vi "PomiarTESTOWYpmp.vi"(3 "Wybór obiektu":u32(slide)=1 scale=1.0..4.0, 4 "WLACZ":bool, 5 "Liniowy/Logarytmiczny":bool, 6 "Amplituda":dbl, 7 "F min":dbl, 8 "ilosc probek":u32, 9 "F max":dbl) -> (0 "Czestotliwosc":dbl[](array[numeric]), 1 "V in":dbl[](array[numeric]), 2 "V out":dbl[](array[numeric]))   [LabVIEW 2021]
doc: "W tym SubVi dokonywany jest pomiar oraz wyliczanę są wymagane wartosci"
uses:
  <userlib>/Open_device_2018.llb/Select_Instr.ctl
panel:
  out "error out 3":errorcluster
  in  "error in (no error) 2":errorcluster
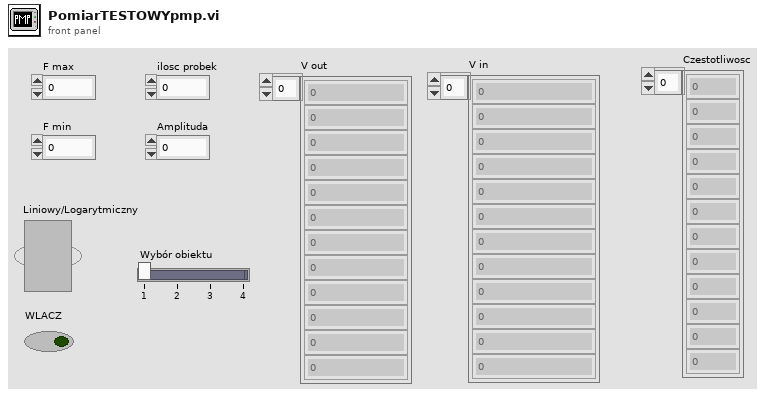
[diagram p1: front panel]
types:
  T1 = typedef "Select_Instr.ctl" = string
  T2 = cluster{"VISA resource name 1":refnum<visa-resource-name>, "VISA resource name 2":refnum<visa-resource-name>, "VISA resource name 3":refnum<visa-resource-name>}
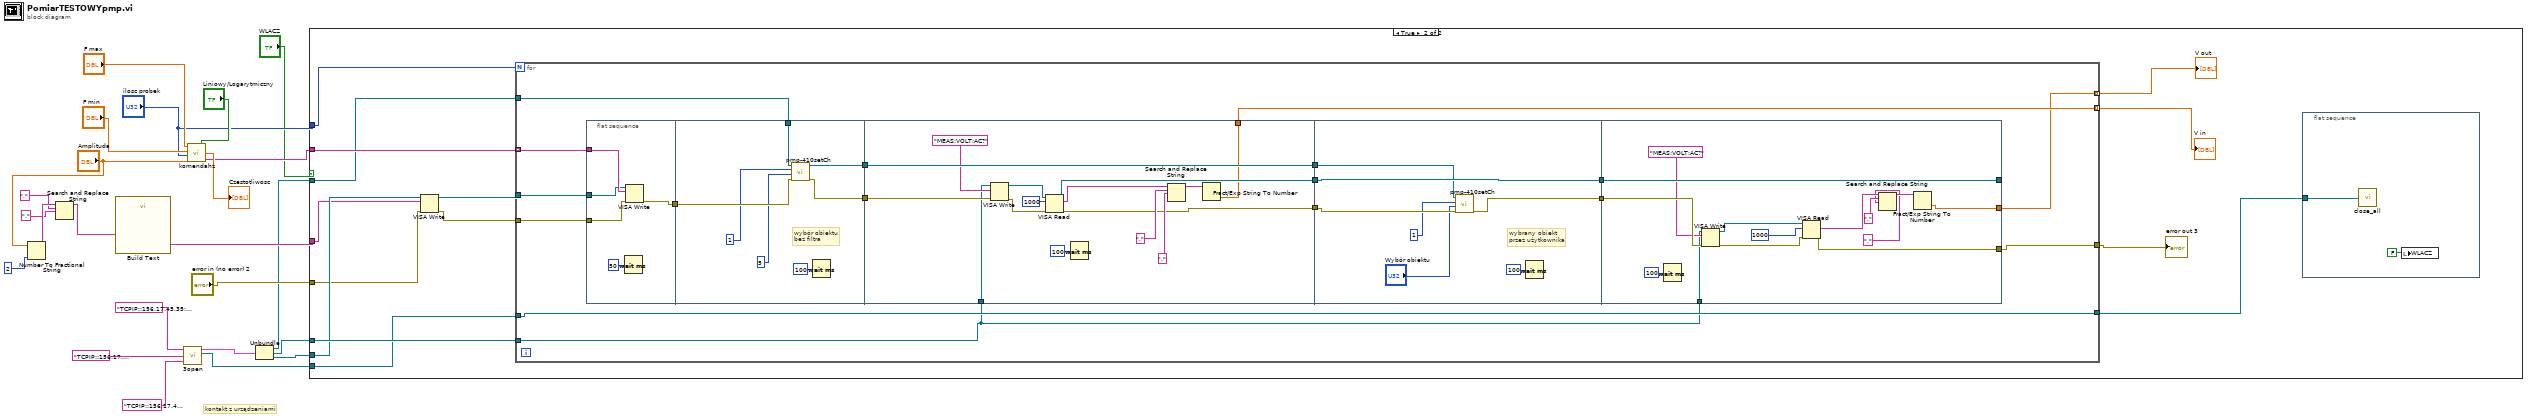
[diagram p0: block diagram]
diagram:
  # "kontakt z urządzeniami"
  n1 = Number To Fractional String(number="Amplituda", precision (6)=i16 2) -> (F-format string=w15:string)  [unwired: 2 in]
  n2 = Search and Replace String(input string=w15, search string=",", replace string="." ("replace string (\"\")")) -> (result string=w12:string)  [unwired: 5 in, 3 out]
  n3 = call "Build Text"("value"=w12) -> ("Result"=w9:string)  [unwired: 13 in, 1 out]
  n4 = call <userlib>:"3open.vi"("VISA resource name 1"=T1 "TCPIP::156.17.45.35::inst104::INSTR" ("Select_Instrument"), "VISA resource name 2"=T1 "TCPIP::156.17.45.35::inst27::INSTR" ("Select_Instrument"), "VISA resource name 3"=T1 "TCPIP::156.17.45.35::inst26::INSTR" ("Select_Instrument")) -> ("InstrCluster"=w5:T2, "InstrArray"=w2:refnum<visa-resource-name>[])  [unwired: 1 in, 2 out]
  n5 = call "komendahz.vi"("Liniowy/logarytmiczny"="Liniowy/Logarytmiczny", "Amplituda"="Amplituda", "ilosc probek"="ilosc probek", "F min"="F min", "F max"="F max") -> ("komendy"=w17:string[], "Czestotliwosci"=→"Czestotliwosc":dbl[])
  n6 = Unbundle(w5) -> ("VISA resource name 1"=w1:refnum<visa-resource-name>, "VISA resource name 2"=w3:refnum<visa-resource-name>, "VISA resource name 3"=w4:refnum<visa-resource-name>)
  n7 = case shown="True" "WLACZ" {
    tunnel: "ilosc probek" -> [_ w37]
    tunnel: "error in (no error) 2" -> [_ w28]
    tunnel: w17 -> [_ w36]
    tunnel: w9 -> [_ w29]
    tunnel: w4 -> [_ w30]
    tunnel: w3 -> [_ w33]
    tunnel: w2 -> [_ w25]
    tunnel: w1 -> [_ w32]
    frame False {
    }
    frame True {
      n8 = VISA Write(VISA resource name=w30, write buffer=w29, error in (no error)=w28) -> (VISA resource name out=w24:refnum<visa-resource-name>, error out=w27:errorcluster)  [unwired: 1 out]
      n9 = for {
        N: w37 -> [_]
        tunnel: w36 -> [w55] mode=indexing
        tunnel: [w41] -> w35 mode=indexing
        tunnel: [w48] -> w34 mode=indexing
        tunnel: w27 -> [w54]
        tunnel: w33 -> [w40]
        tunnel: w32 -> [w51]
        tunnel: [w56] -> w31
        tunnel: w25 -> [w56]
        tunnel: [w42] -> w26
        tunnel: w24 -> [w53]
        n10 = flat-sequence {
          tunnel: w55 -> [w61]
          tunnel: w54 -> [w60]
          tunnel: w53 -> [w58]
          tunnel: [w59] -> w52
          tunnel: w52 -> [w68]
          tunnel: w51 -> [w65]
          tunnel: [w64] -> w50
          tunnel: [w63] -> w49
          tunnel: w50 -> [w77]
          tunnel: w49 -> [w83]
          tunnel: w40 -> [w75]
          tunnel: [w70] -> w48
          tunnel: [w83] -> w47
          tunnel: [w72] -> w46
          tunnel: [w71] -> w45
          tunnel: w47 -> [w87]
          tunnel: w46 -> [w89]
          tunnel: w45 -> [w90]
          tunnel: [w90] -> w44
          tunnel: [w86] -> w43
          tunnel: [w104] -> _
          tunnel: w44 -> [w104]
          tunnel: w43 -> [w98]
          tunnel: [w94] -> w42
          tunnel: [w93] -> w41
          tunnel: w40 -> [w91]
          frame #0 {
            n11 = Wait (ms)(milliseconds to wait=u32 50) -> ()  [unwired: 1 out]
            n12 = VISA Write(VISA resource name=w58, write buffer=w61, error in (no error)=w60) -> (error out=w59:errorcluster)  [unwired: 2 out]
          }
          frame #1 {
            # "wybór obiektu\nbez filtra"
            n13 = call <userlib>:"pmp-410setCh.vi"("error in (no error)"=w68, "Channel"=u8 5, "Slave#"=u8 1, "VISA Refnum in"=w65) -> ("error out"=w64:errorcluster, "VISA Refnum out"=w63:refnum<visa-resource-name>)  [unwired: 6 in]
            n14 = Wait (ms)(milliseconds to wait=u32 100) -> ()  [unwired: 1 out]
          }
          frame #2 {
            n15 = VISA Write(VISA resource name=w75, write buffer="MEAS:VOLT:AC?", error in (no error)=w77) -> (VISA resource name out=w80:refnum<visa-resource-name>, error out=w81:errorcluster)  [unwired: 1 out]
            n16 = VISA Read(VISA resource name=w80, byte count=u32 1000, error in (no error)=w81) -> (VISA resource name out=w71:refnum<visa-resource-name>, read buffer=w82:string, error out=w72:errorcluster)  [unwired: 1 out]
            n17 = Wait (ms)(milliseconds to wait=u32 100) -> ()  [unwired: 1 out]
            n18 = Search and Replace String(input string=w82, search string=".", replace string="," ("replace string (\"\")")) -> (result string=w79:string)  [unwired: 5 in, 3 out]
            n19 = Fract/Exp String To Number(string=w79) -> (number=w70:dbl)  [unwired: 3 in, 1 out]
          }
          frame #3 {
            # "wybrany obiekt\nprzez użytkownika"
            n20 = call <userlib>:"pmp-410setCh.vi"("error in (no error)"=w89, "Channel"="Wybór obiektu", "Slave#"=u8 1, "VISA Refnum in"=w87) -> ("error out"=w86:errorcluster)  [unwired: 6 in, 1 out]
            n21 = Wait (ms)(milliseconds to wait=u32 100) -> ()  [unwired: 1 out]
          }
          frame #4 {
            n22 = Wait (ms)(milliseconds to wait=u32 100) -> ()  [unwired: 1 out]
            n23 = VISA Write(VISA resource name=w91, write buffer="MEAS:VOLT:AC?", error in (no error)=w98) -> (VISA resource name out=w101:refnum<visa-resource-name>, error out=w102:errorcluster)  [unwired: 1 out]
            n24 = VISA Read(VISA resource name=w101, byte count=u32 1000, error in (no error)=w102) -> (read buffer=w103:string, error out=w94:errorcluster)  [unwired: 2 out]
            n25 = Search and Replace String(input string=w103, search string=".", replace string="," ("replace string (\"\")")) -> (result string=w100:string)  [unwired: 5 in, 3 out]
            n26 = Fract/Exp String To Number(string=w100) -> (number=w93:dbl)  [unwired: 3 in, 1 out]
          }
        }
      }
      "V out" <- w35
      "V in" <- w34
      "error out 3" <- w26
      n27 = flat-sequence {
        tunnel: w31 -> [w38]
        frame #0 {
          n28 = call <userlib>:"close_all.vi"("OpenRes"=w38) -> ()  [unwired: 1 out]
          n29 = local write "WLACZ"(FALSE ("WLACZ")) -> ()
        }
      }
    }
  }
